vi "new Control rack controller.vi"() -> ()   [LabVIEW 2011]
uses:
  <vilib>/DAQmx/write.llb/DAQmx Write (Analog DBL 1Chan 1Samp).vi
  <vilib>/DAQmx/create/channels.llb/DAQmx Create Channel (AO-Voltage-Basic).vi
  <vilib>/DAQmx/miscellaneous.llb/DAQmx Fill In Error Info.vi
panel:
  in  "Voltages Toroidal (Keep below |10|)":dbl[](array[numeric])
  out "Current Voltage Toroidal":dbl
  in  "Timestep (in seconds, keep above 1/20s)":dbl
  in  "Voltages Helical (Keep below |10|)":dbl[](array[numeric])
  in  "Times":dbl[](array[numeric])
  out "Current Time":dbl
  out "Current Voltage Helical":dbl
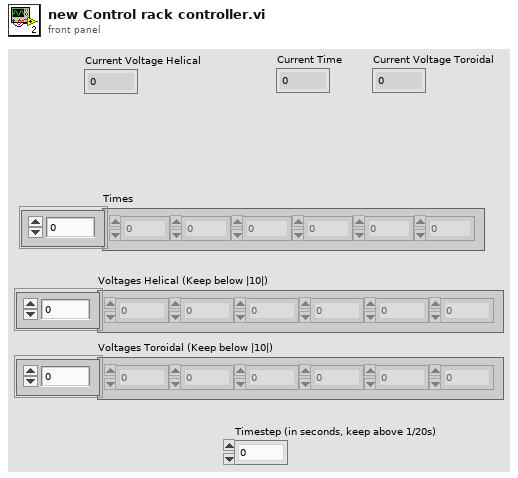
[diagram p1: front panel]
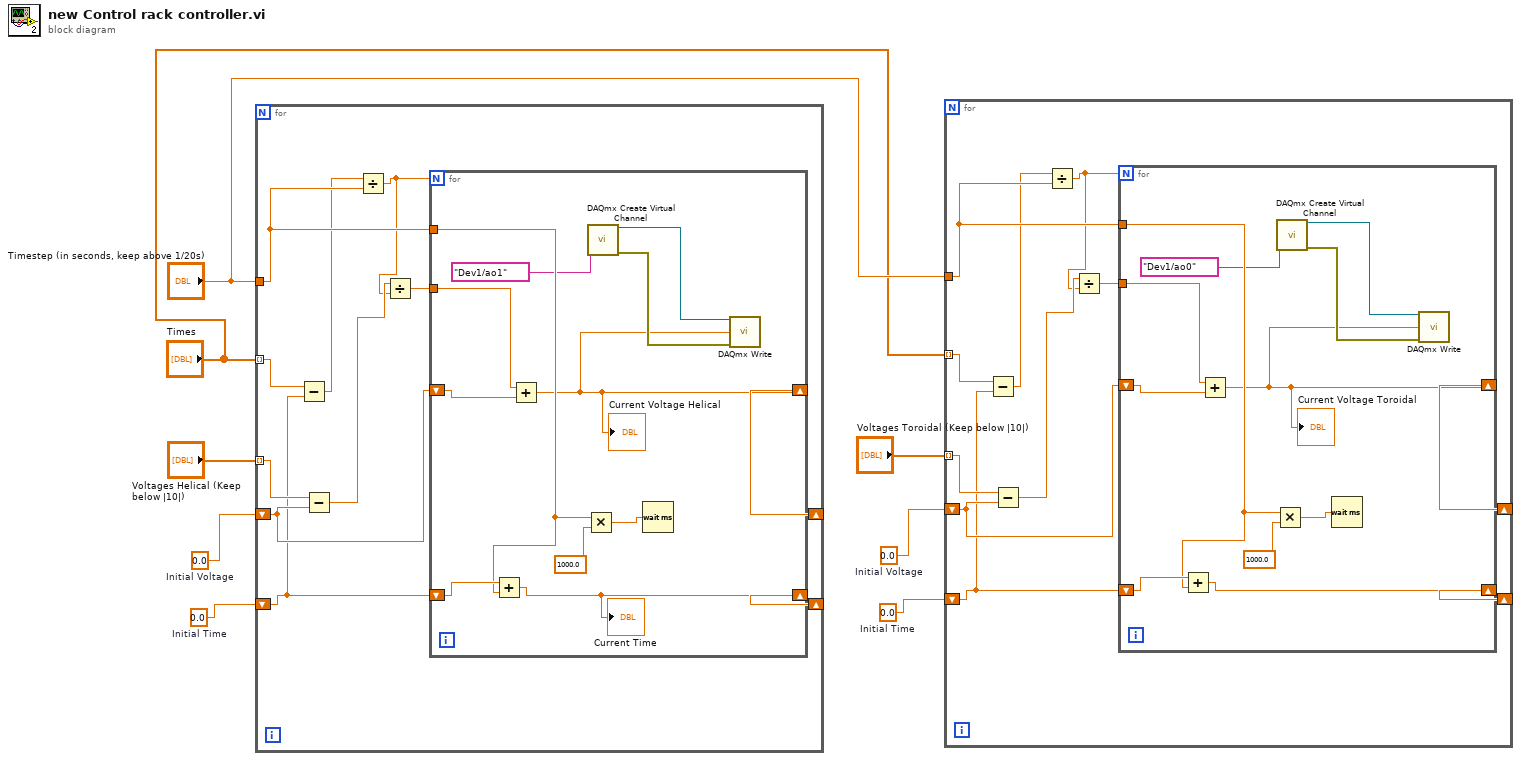
[diagram p0: block diagram]
diagram:
  w5 = 0.0  # Initial Time
  w4 = 0.0  # Initial Voltage
  w6 = 0.0  # Initial Time
  w7 = 0.0  # Initial Voltage
  n1 = for {
    tunnel: "Voltages Helical (Keep below |10|)" -> [w19] mode=indexing
    tunnel: "Times" -> [w12] mode=indexing
    tunnel: "Timestep (in seconds, keep above 1/20s)" -> [w14]
    shift-right: [w15] -> _
    shift-left: w7 -> [w18]
    shift-right: [w13] -> _
    shift-left: w6 -> [w11]
    n2 = Subtract(x=w12, y=w11) -> (x-y=w10:dbl)
    n3 = Subtract(x=w19, y=w18) -> (x-y=w17:dbl)
    n4 = Divide(x=w10, y=w14) -> (x/y=w9:dbl)
    n5 = Divide(x=w17, y=w9) -> (x/y=w16:dbl)
    n6 = for {
      N: w9 -> [_]
      shift-right: [w20] -> w15
      shift-left: w18 -> [w30]
      tunnel: w16 -> [w29]
      tunnel: w14 -> [w26]
      shift-right: [w24] -> w13
      shift-left: w11 -> [w28]
      n7 = Add(x=w28, y=w26) -> (x+y=w24:dbl)
      "Current Time" <- w24
      n8 = Add(x=w29, y=w30) -> (x+y=w20:dbl)
      "Current Voltage Helical" <- w20
      n9 = Multiply(x=w26, y=1000.0) -> (x*y=w27:dbl)
      n10 = call-poly <vilib>:"DAQmx Create Virtual Channel.vi"("physical channels"=tag "Dev1/ao1" ("write channel (torr = ao0, hel = ao1)")) -> ("task out"=w21:refnum<k21>, "error out"=w22:errorcluster)  [unwired: 13 in]
      n11 = Wait (ms)(milliseconds to wait=w27) -> ()  [unwired: 1 out]
      n12 = call-poly <vilib>:"DAQmx Write.vi"("task/channels in"=w21, "data"=w20, "error in"=w22) -> ()  [unwired: 10 in, 3 out]
    }
  }
  n13 = for {
    tunnel: "Voltages Toroidal (Keep below |10|)" -> [w41] mode=indexing
    tunnel: "Times" -> [w34] mode=indexing
    tunnel: "Timestep (in seconds, keep above 1/20s)" -> [w36]
    shift-right: [w37] -> _
    shift-left: w4 -> [w40]
    shift-right: [w35] -> _
    shift-left: w5 -> [w33]
    n14 = Subtract(x=w34, y=w33) -> (x-y=w32:dbl)
    n15 = Subtract(x=w41, y=w40) -> (x-y=w39:dbl)
    n16 = Divide(x=w32, y=w36) -> (x/y=w31:dbl)
    n17 = Divide(x=w39, y=w31) -> (x/y=w38:dbl)
    n18 = for {
      N: w31 -> [_]
      shift-right: [w42] -> w37
      shift-left: w40 -> [w52]
      tunnel: w38 -> [w51]
      tunnel: w36 -> [w48]
      shift-right: [w46] -> w35
      shift-left: w33 -> [w50]
      n19 = Add(x=w50, y=w48) -> (x+y=w46:dbl)
      n20 = Add(x=w51, y=w52) -> (x+y=w42:dbl)
      "Current Voltage Toroidal" <- w42
      n21 = Multiply(x=w48, y=1000.0) -> (x*y=w49:dbl)
      n22 = call-poly <vilib>:"DAQmx Create Virtual Channel.vi"("physical channels"=tag "Dev1/ao0" ("write channel (torr = ao0, hel = ao1) 2")) -> ("task out"=w43:refnum<k21>, "error out"=w44:errorcluster)  [unwired: 13 in]
      n23 = Wait (ms)(milliseconds to wait=w49) -> ()  [unwired: 1 out]
      n24 = call-poly <vilib>:"DAQmx Write.vi"("task/channels in"=w43, "data"=w42, "error in"=w44) -> ()  [unwired: 10 in, 3 out]
    }
  }
